vi "CalculateAngleDistance.vi"(10 "Current Position":dbl, 11 "Desired Position":dbl) -> (3 "Distance":dbl)   [LabVIEW 2016]
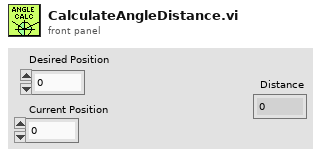
[diagram p1: front panel]
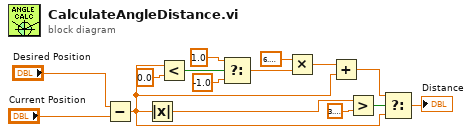
[diagram p0: block diagram]
diagram:
  n1 = Subtract(x="Desired Position", y="Current Position") -> (x-y=w1:dbl)
  n2 = Absolute Value(x=w1) -> (abs(x)=w12:dbl)
  n3 = Less?(x=w1, y=0.0) -> (x < y?=w10:bool)
  n4 = Select(t=1.0, s=w10, f=-1.0) -> (s? t:f=w5:dbl)
  n5 = Multiply(x=6.283185307179586, y=w5) -> (x*y=w4:dbl)
  n6 = Add(x=w4, y=w1) -> (x+y=w3:dbl)
  n7 = Greater?(x=w12, y=3.141592653589793) -> (0:w13:bool)
  n8 = Select(t=w3, s=w13, f=w1) -> (s? t:f=→"Distance":dbl)
